vi "Exit Event Loop.vi"(8 "error in (no error)":errorcluster, 11 "GUI Container Actor in":refnum<class "GUI Container Actor.lvclass">) -> (0 "error out":errorcluster, 3 "GUI Container Actor out":refnum<class "GUI Container Actor.lvclass">)   [LabVIEW 2017, in "GUI Views.lvlib" / "GUI Container Actor.lvclass"]
doc: "This method must be used in the Actor Core of the subclass of the GUI Container Actor. If in this acotr core the method Register to View Event was called and the helper event loop is listening to the corresponding event calling this method will cause the helper event loop to exit. This is useful to allow the exit of the helper loop when the stop bessage of the actor is received. Calling this method is optional. See the examples for an illustration of its usage"
uses:
  GUI Container Actor.lvclass
  GUI Container Actor.lvclass/GUI Container Actor.ctl
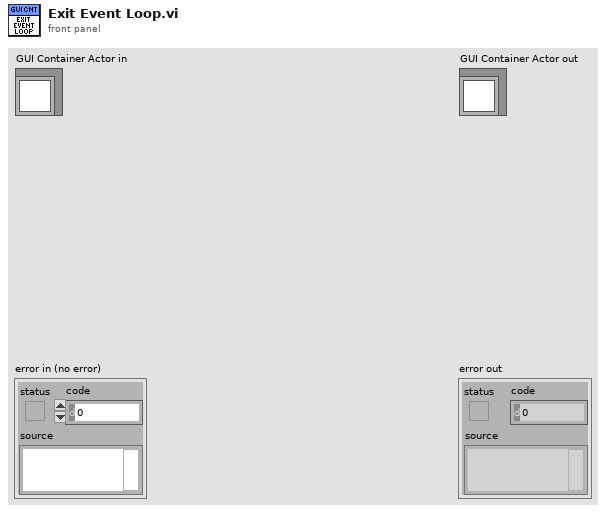
[diagram p1: front panel]
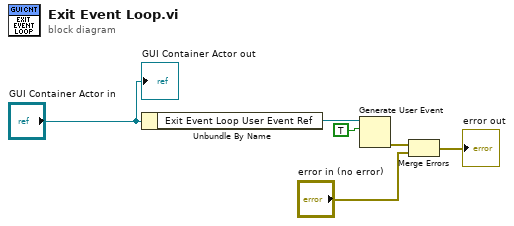
[diagram p0: block diagram]
diagram:
  n1 = Unbundle By Name("GUI Container Actor in") -> ("Exit Event Loop User Event Ref"=w4:refnum<user-event>)
  n2 = Generate User Event(user event=w4, event data cluster=TRUE ("event data")) -> (error out=w1:errorcluster)  [unwired: 2 in, 1 out]
  n3 = Merge Errors(w1, "error in (no error)") -> (→"error out":errorcluster)
  "GUI Container Actor out" <- "GUI Container Actor in"
